vi "1 Channel N Samples - Manual Timestamps.vi"() -> ()   [LabVIEW 2026, in "synnax_clib.lvlib"]
uses:
  lvlib/typedefs/connection_config.ctl
  lvlib/classes/Client/Private/synnax channel retrieve keys Single.vi
  lvlib/classes/Writer/Private/synnax writer open Array.vi
  lvlib/classes/Writer/Private/Writes/DBL/Write 1Ch NSamp (DBL).vi
  lvlib/synnax_clib.lvlib
  lvlib/classes/Synnax Writer.lvclass
  lvlib/classes/Client/Synnax Client.lvclass
panel:
  in  "Channel":string="my_f64_chan"
  in  "Stop":bool
  out "error out":errorcluster
  in  "Connection Config":T1={"host"="localhost", "port"=9090, "username"="synnax", "password"="seldon"}
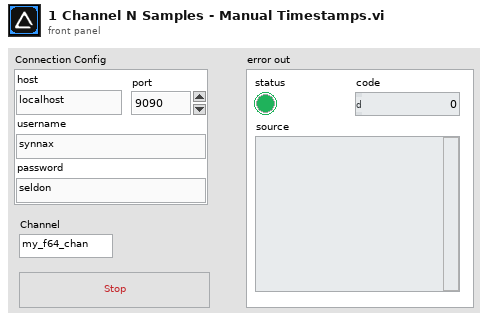
[diagram p1: front panel]
types:
  T1 = typedef "synnax_clib.lvlib/connection_config.ctl" = cluster{"host":string, "port":u16, "username":string, "password":string}
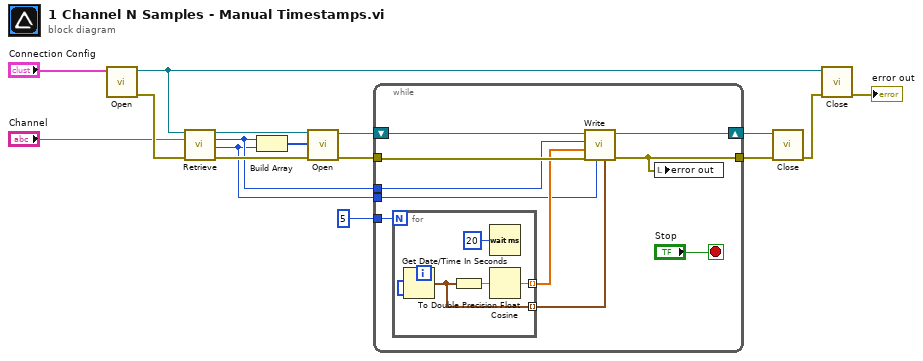
[diagram p0: block diagram]
diagram:
  n1 = call "Open.vi"("Connection Config"="Connection Config") -> ("error out"=w11:errorcluster, "Synnax Client out"=w13:refnum<class "Synnax Client.lvclass">)  [unwired: 9 in]
  n2 = call-poly "Retrieve.vi"("Synnax Client in"=w13, "channel name"="Channel", "error in"=w11) -> ("Synnax Client out"=w7:refnum<class "Synnax Client.lvclass">, "channel key"=w3:u32, "index key"=w2:u32, "error out"=w15:errorcluster)  [unwired: 8 in, 1 out]
  n3 = Build Array(w3, w2) -> (w4:u32[])
  n4 = call-poly "Open.vi"("error in"=w15, "channels in"=w4, "Synnax Client in"=w7) -> ("error out"=w8:errorcluster, "writer out"=w10:refnum<class "Synnax Writer.lvclass">)  [unwired: 6 in, 1 out]
  n5 = while {
    shift-right: [w25] -> w9
    shift-left: w10 -> [w26]
    tunnel: w8 -> [w24]
    tunnel: [w21] -> w16
    tunnel: w2 -> [w20]
    tunnel: w3 -> [w18]
    tunnel: 5 -> [w17]
    stop <- "Stop" stop-if-true
    n6 = for {
      N: w17 -> [_]
      tunnel: [w30] -> w22 mode=indexing
      tunnel: [w28] -> w19 mode=indexing
      n7 = Get Date/Time In Seconds() -> (seconds since 1Jan1904=w28:timestamp)
      n8 = To Double Precision Float(number=w28) -> (double precision float=w29:dbl)
      n9 = Wait (ms)(milliseconds to wait=u32 20) -> ()  [unwired: 1 out]
      n10 = Cosine(x=w29) -> (cos(x)=w30:dbl)
    }
    n11 = call-poly "Write.vi"("timestamps"=w19, "index_channel"=w20, "error in"=w24, "data"=w22, "channel"=w18, "Writer"=w26) -> ("error out"=w21:errorcluster, "Writer Out"=w25:refnum<class "Synnax Writer.lvclass">)  [unwired: 4 in]
    n12 = local write "error out"(w21) -> ()
  }
  n13 = call "Close.vi"("error in"=w16, "writer"=w9) -> ("error out"=w12:errorcluster)  [unwired: 9 in]
  n14 = call "Close.vi"("error in"=w12, "Synnax Client in"=w13) -> ("error out"=→"error out":errorcluster)  [unwired: 9 in]
